vi "SaveScannedNodes.vi"(11 "Scanned Nodes":T1 {"Year" format="%02d"; "Patient Number" format="%03d"; "Node Number" format="%02d"}) -> ()   [LabVIEW 2022 SP3]
uses:
  ScannedNodeArray.ctl
  LymphNodeInfo.ctl
  TissueTypeScan.ctl
  PatientGlobals.vi
  <vilib>/Utility/xml.llb/Write to XML File(string).vi
panel:
  out "error out":errorcluster
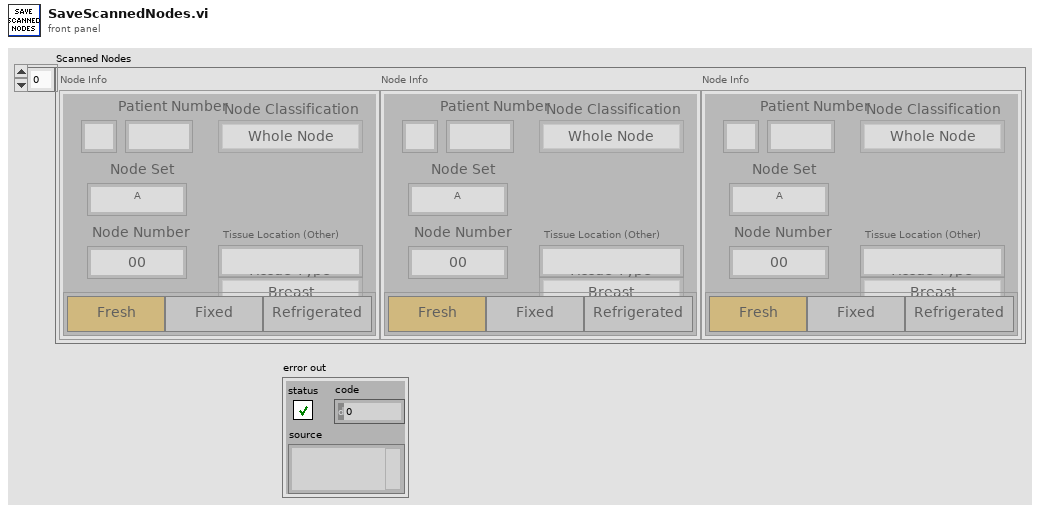
[diagram p1: front panel]
types:
  T1 = typedef "ScannedNodeArray.ctl" = T2[]
  T2 = typedef "LymphNodeInfo.ctl" = cluster{"Patient Number":u32, "Node Set":string, "Node Number":u32, "Tissue Type":T3, "Tissue Location (Other)":string, "Node Classification":enum16{"Whole Node", "Piece A", "Piece B", "Piece C"}, "Fresh?":enum32{"Fresh?", "Fixed?", "Refrigerated?"}, "Year":u32}
  T3 = typedef "TissueTypeScan.ctl" = enum16{"Breast", "Gastric", "Stomach", "Rectal", "Colon", "Head & Neck", "Other"}
  T4 = enum16{"open", "replace", "create", "open or create", "replace or create", "replace or create with confirmation"}
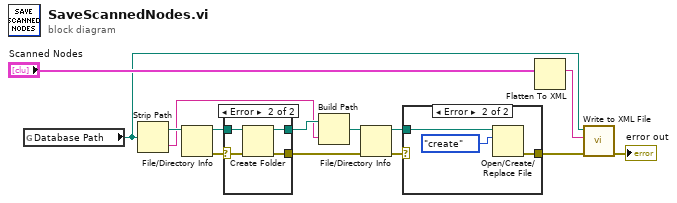
[diagram p0: block diagram]
diagram:
  n1 = global read "PatientGlobals.vi" "Database Path"() -> (w9:path)
  n2 = Strip Path(path=w9) -> (stripped path=w8:path, name=w2:string)
  n3 = File/Directory Info(path=w8) -> (path out=w7:path, error out=w6:errorcluster)  [unwired: 1 in, 5 out]
  n4 = case shown="Error" w6 {
    selector: w6 -> [w16 w18]
    tunnel: w7 -> [w15 w20]
    tunnel: [w16 w19] -> w5
    tunnel: [w15 w17] -> w3
    frame No Error {
    }
    frame Error {
      n5 = Create Folder(path (use dialog)=w20, error in=w18) -> (created path=w17:path, error out=w19:errorcluster)  [unwired: 2 out]
    }
  }
  n6 = Build Path(base path=w3, name or relative path=w2) -> (appended path=w1:path)
  n7 = File/Directory Info(path=w1, error in=w5) -> (path out=w11:path, error out=w12:errorcluster)  [unwired: 5 out]
  n8 = case shown="Error" w12 {
    selector: w12 -> [w21 _]
    tunnel: w11 -> [_ w24]
    tunnel: [w21 w23] -> w10
    frame No Error {
    }
    frame Error {
      n9 = Open/Create/Replace File(file path (use dialog)=w24, operation (0:open)=T4."create") -> (error out=w23:errorcluster)  [unwired: 4 in, 2 out]
    }
  }
  n10 = Flatten To XML(6:"Scanned Nodes") -> (2:w14:string)
  n11 = call-poly <vilib>:"Write to XML File.vi"("error in (no error)"=w10, "XML Input"=w14, "XML File Path"=w9) -> ("error out"=→"error out":errorcluster)  [unwired: 6 in, 2 out]
